vi "MainPane SubView Exit.vi"(8 "error in (no error)":errorcluster, 11 "MainController in":refnum<class "MainController.lvclass">) -> (0 "error out":errorcluster, 3 "MainController out":refnum<class "MainController.lvclass">)   [LabVIEW 2012, in "Win8uiFramework.lvlib" / "MainController.lvclass"]
uses:
  MainController.lvclass
  Slide Direction.ctl
  Win8uiFramework.lvlib
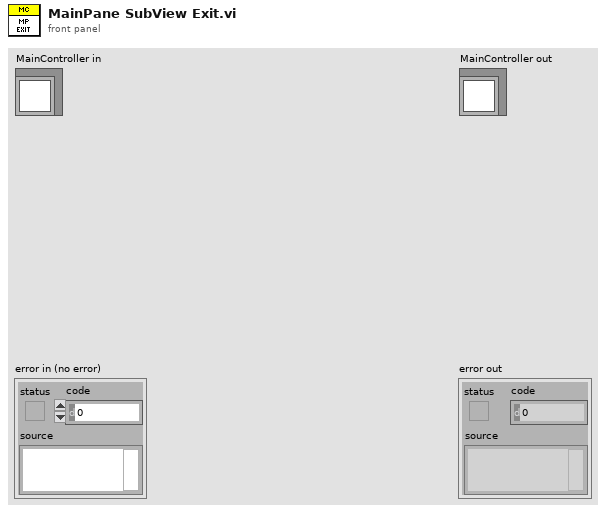
[diagram p1: front panel]
types:
  T1 = typedef "Win8uiFramework.lvlib/Slide Direction.ctl" = enum16{"Forwards", "Back"}
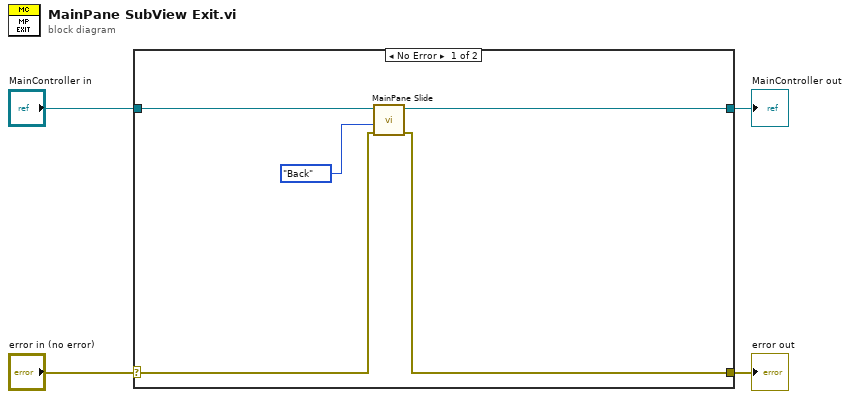
[diagram p0: block diagram]
diagram:
  n1 = case shown="No Error" "error in (no error)" {
    selector: "error in (no error)" -> [w6 w11]
    tunnel: [w5 w11] -> w3
    tunnel: [w8 w10] -> w1
    tunnel: "MainController in" -> [w9 w10]
    frame No Error {
      n2 = call-dynamic "MainPane Slide.vi"("error in (no error)"=w6, "Slide Direction"=Slide_Direction."Back", "MainController in"=w9) -> ("error out"=w5:errorcluster, "MainController out"=w8:refnum<class "MainController.lvclass">)  [unwired: 7 in]
    }
    frame Error {
    }
  }
  "error out" <- w3
  "MainController out" <- w1
